vi "Shoot_Command.vi"   [LabVIEW 2014]
uses:
  TORC Code/GlobalVariable.vi
types:
  T1 = enum16{"Unready", "Ready", "Clear", "Fire", "Reload", "Arm In"}
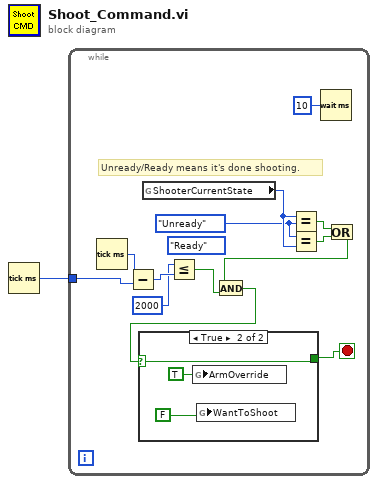
[diagram p0: block diagram]
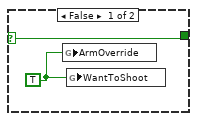
[diagram p2: hidden frame]
diagram:
  n1 = Tick Count (ms)() -> (millisecond timer value=w1:u32)
  n2 = while {
    tunnel: w1 -> [w4]
    stop <- w7 stop-if-true
    (unwired) T1."Ready" ("y")
    w11 = T1."Unready" ("y")
    # "Unready/Ready means it's done shooting."
    n3 = Tick Count (ms)() -> (millisecond timer value=w5:u32)
    n4 = Subtract(x=w5, y=w4) -> (x-y=w6:u32)
    n5 = global read "GlobalVariable.vi" "ShooterCurrentState"() -> (w12:T1)
    n6 = Less Or Equal?(x=u32 2000 ("Delay ms"), y=w6) -> (x <= y?=w2:bool)
    n7 = Equal?(x=w12, y=w11) -> (x = y?=w13:bool)
    n8 = Equal?(x=w11, y=w12) -> (x = y?=w10:bool)
    n9 = Wait (ms)(milliseconds to wait=u32 10) -> ()  [unwired: 1 out]
    n10 = Or(x=w13, y=w10) -> (x .or. y?=w9:bool)
    n11 = And(x=w9, y=w2) -> (x .and. y?=w8:bool)
    n12 = case shown="True" w8 {
      selector: w8 -> [w15 w18]
      tunnel: [w15 w18] -> w7
      frame False {
        w16 = TRUE ("WantToShoot")
        n13 = global write "GlobalVariable.vi" "ArmOverride"(w16) -> ()
        n14 = global write "GlobalVariable.vi" "WantToShoot"(w16) -> ()
      }
      frame True {
        n15 = global write "GlobalVariable.vi" "ArmOverride"(TRUE ("ArmOverride")) -> ()
        n16 = global write "GlobalVariable.vi" "WantToShoot"(FALSE ("WantToShoot")) -> ()
      }
    }
  }
